vi "makeNewDirectory.vi"(9 "error in (no error)":errorcluster, 10 "path":path) -> (1 "error out":errorcluster, 2 "path out":path)   [LabVIEW 2010]
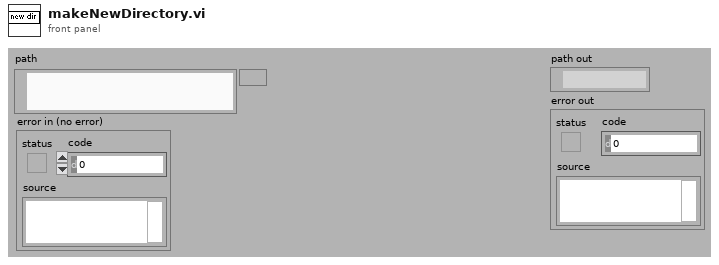
[diagram p1: front panel]
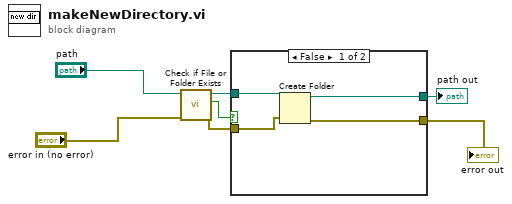
[diagram p0: block diagram]
diagram:
  n1 = call <vilib>:"Check if File or Folder Exists.vi"("error in (no error)"="error in (no error)", "path"="path") -> ("error out"=w4:errorcluster, "file or folder exists?"=w6:bool, "dup path"=w5:path)  [unwired: 7 in]
  n2 = case shown="False" w6 {
    tunnel: w5 -> [w11 w13]
    tunnel: [w10 w13] -> w2
    tunnel: w4 -> [w9 w12]
    tunnel: [w8 w12] -> w1
    frame False {
      n3 = Create Folder(path (use dialog)=w11, error in=w9) -> (created path=w10:path, error out=w8:errorcluster)  [unwired: 1 in, 1 out]
    }
    frame True {
    }
  }
  "path out" <- w2
  "error out" <- w1
